vi "Read Waveform Measurement (Time).vi"(0 "VISA resource name":refnum<visa-resource-name>, 1 "Maximum Time (25000ms)":u32=25000, 5 "Channel1 (0:Channel1)":u16(ring) items=["Channel1", "Channel2", "Channel3", "Channel4", "Math1", "Math2", "Math3", "Math3", "Reference1", "Reference2", "Reference3", "Reference4"], 7 "Function (0:Rise Time)":u16(ring) items=["Rise Time", "Pos Width", "Period", "Fall Time", "Neg Width", "Frequency", "+Duty Cycle", "-Duty Cycle", "Delay"], 9 "Channel2 (1:Channel2)":u16(ring)=1 items=["Channel1", "Channel2", "Channel3", "Channel4", "Math1", "Math2", "Math3", "Math3", "Reference1", "Reference2", "Reference3", "Reference4"], 11 "error in (no error)":errorcluster, 12 "Search Direction (0:Forward)":u16(ring) items=["Forward", "Backwards"], 13 "Delay Edge1 (0:Rise Time)":u16(ring) items=["Rise Time", "Fall Time "], 14 "Delay Edge2 (0:Rise Time)":u16(ring) items=["Rise Time", "Fall Time"]) -> (4 "VISA resource name out":refnum<visa-resource-name>, 6 "Measurement":dbl, 15 "error out":errorcluster)   [LabVIEW 2015, in "Tektronix 7000 Series.lvlib"]
doc: "Initiates an acquisition on the channels that you enable with the Configure Channel VI. This VI then waits for the acquisition to complete, obtains a waveform measurement on the channels you specify, and returns the measurement value."
uses:
  <instrlib>/Tektronix 7000 Series/Tektronix 7000 Series.lvlib
  <instrlib>/Tektronix 7000 Series/Public/Data/Low Level/Fetch Waveform Measurement (Time).vi
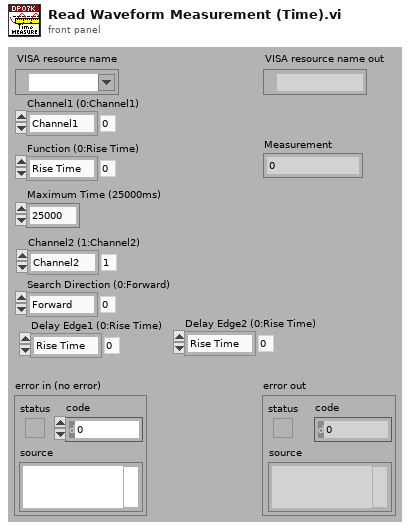
[diagram p1: front panel]
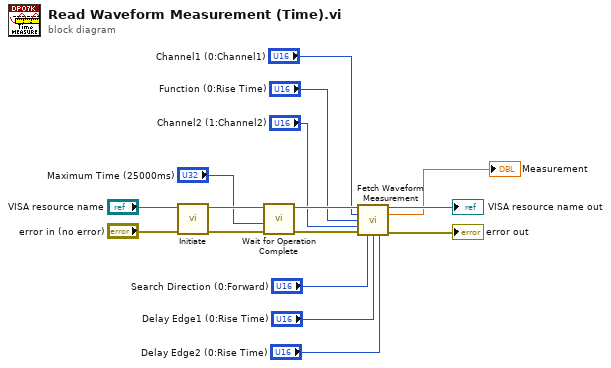
[diagram p0: block diagram]
diagram:
  n1 = call <instrlib>:"Initiate.vi"("error in (no error)"="error in (no error)", "VISA resource name"="VISA resource name") -> ("error out"=w16:errorcluster, "VISA resource name out"=w15:refnum<visa-resource-name>)  [unwired: 8 in]
  n2 = call <instrlib>:"Wait for Operation Complete.vi"("error in (no error)"=w16, "Maximum Time (2000ms)"="Maximum Time (25000ms)", "VISA resource name"=w15) -> ("error out"=w9:errorcluster, "VISA resource name out"=w10:refnum<visa-resource-name>)  [unwired: 7 in]
  n3 = call-poly <instrlib>:"Fetch Waveform Measurement.vi"("VISA resource name"=w10, "Channel A (0:Channel 1)"="Channel1 (0:Channel1)", "Function (0:Rise Time)"="Function (0:Rise Time)", "Channel B (1:Channel 2)"="Channel2 (1:Channel2)", "error in (no error)"=w9, "Search Direction (0:Forward)"="Search Direction (0:Forward)", "Delay Edge1 (0:Rise Time)"="Delay Edge1 (0:Rise Time)", "Delay Edge2 (0:Rise Time)"="Delay Edge2 (0:Rise Time)") -> ("VISA resource name out"=→"VISA resource name out":refnum<visa-resource-name>, "Measurement"=→"Measurement":dbl, "error out"=→"error out":errorcluster)  [unwired: 5 in]
